vi "Soft Limits.vi"(8 "Input":dbl, 9 "String Pot":dbl, 10 "Reverse Soft Limit":dbl, 11 "Forwards Soft Limit":dbl) -> (3 "Output":dbl)   [LabVIEW 2014]
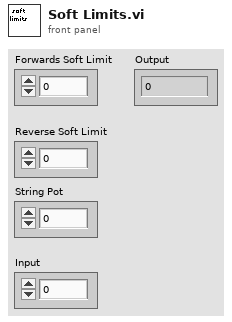
[diagram p1: front panel]
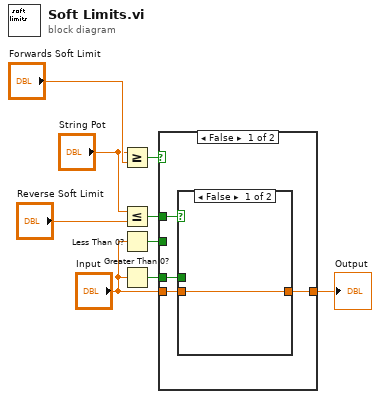
[diagram p0: block diagram]
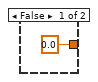
[diagram p3: hidden frame]
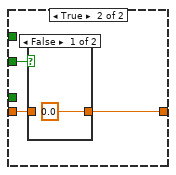
[diagram p4: hidden frame]
diagram:
  n1 = Greater Or Equal?(x="String Pot", y="Forwards Soft Limit") -> (x >= y?=w6:bool)
  n2 = Less Or Equal?(x="String Pot", y="Reverse Soft Limit") -> (x <= y?=w3:bool)
  n3 = Less Than 0?(x="Input") -> (x < 0?=w5:bool)
  n4 = Greater Than 0?(x="Input") -> (x > 0?=w1:bool)
  n5 = case shown="False" w6 {
    tunnel: w5 -> [_ w22]
    tunnel: "Input" -> [w11 w21]
    tunnel: [w10 w20] -> w4
    tunnel: w3 -> [w13 _]
    tunnel: w1 -> [w12 _]
    frame False {
      n6 = case shown="False" w13 {
        tunnel: w12 -> [_ w17]
        tunnel: w11 -> [w14 w16]
        tunnel: [w14 w15] -> w10
        frame False {
        }
        frame True {
          n7 = case shown="True" w17 {
            tunnel: w16 -> [_ w19]
            tunnel: [0.0 ("Input") w19] -> w15
            frame False {
            }
            frame True {
            }
          }
        }
      }
    }
    frame True {
      n8 = case shown="False" w22 {
        tunnel: w21 -> [_ w24]
        tunnel: [0.0 ("Input") w24] -> w20
        frame False {
        }
        frame True {
        }
      }
    }
  }
  "Output" <- w4
